vi "Get Status.vi"(7 "Server Alias":string, 8 "error in (no error)":errorcluster, 9 "Clear Status? (F)":bool, 10 "Include Script Status? (T)":bool=TRUE, 11 "Include Timestamps in Script Status? (T)":bool=TRUE) -> (0 "error out":errorcluster, 1 "Script Status":string, 2 "Connected":bool, 4 "All Scripts":T1[](array[typedef]), 5 "Python Just Disconnected":bool, 6 "Index of Last Line":i32)   [LabVIEW 2013, in "TS.lvlib"]
doc: "This VI polls the Server to know the status, whether the LV side is initialized, whether there is a connection with the Python side, and the status of any scripts running."
uses:
  TS.lvlib
  Private/Status Message.ctl
  LabVIEW Example/Supporting Code/Script Running.ctl
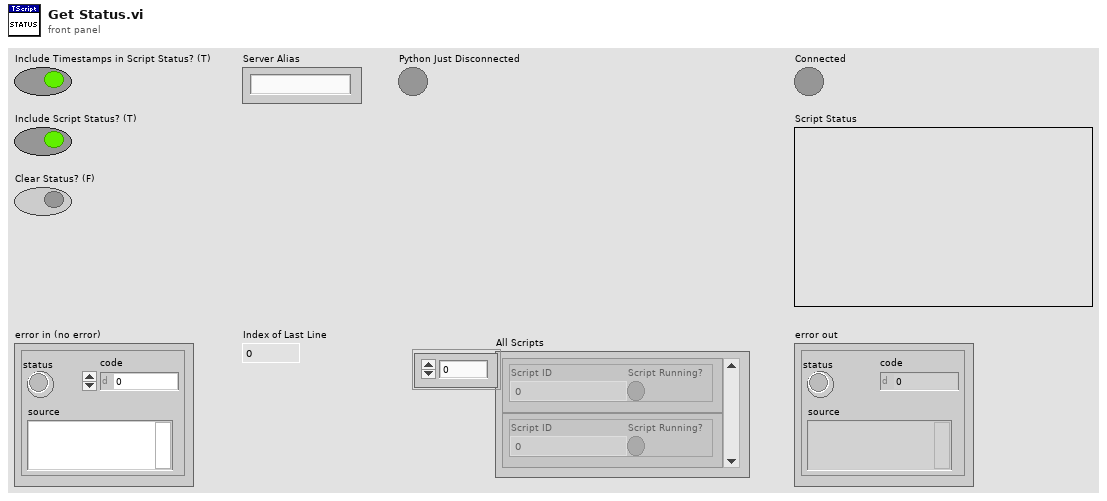
[diagram p1: front panel]
types:
  T1 = typedef "TS.lvlib/Script Running.ctl" = cluster{"Script ID":i64, "Script Running?":bool}
  T2 = typedef "TS.lvlib/Status Message.ctl" = cluster{"Text":string, "Time":timestamp}
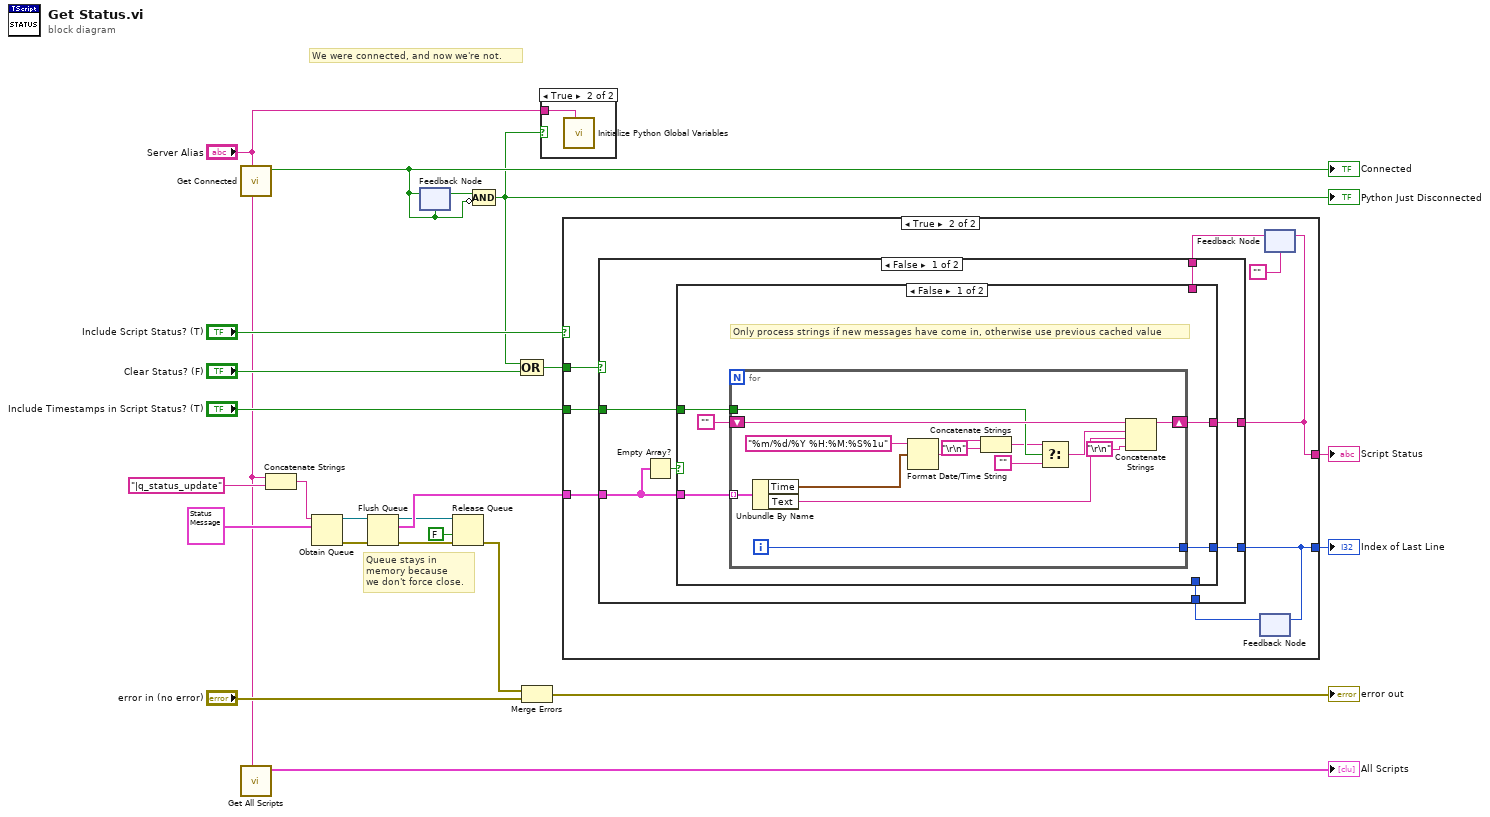
[diagram p0: block diagram]
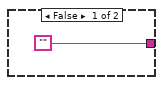
[diagram p3: hidden frame]
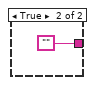
[diagram p5: hidden frame]
diagram:
  # "Queue stays in \nmemory because\nwe don't force close."
  # "We were connected, and now we're not."
  n1 = call "Get Connected.vi"("Server Alias"="Server Alias") -> ("Connected"=w4:bool)  [unwired: 9 in, 1 out]
  "Connected" <- w4
  n2 = call "Get All Scripts.vi"("Server Alias"="Server Alias") -> ("All Scripts"=→"All Scripts":T1[])  [unwired: 9 in, 1 out]
  n3 = Concatenate Strings("Server Alias", "|q_status_update" ("name (unnamed)")) -> (w3:string)
  n4 = Obtain Queue(name (unnamed)=w3, element data type=T2 {"Text"="", "Time"=timestamp(0 s since 1904-01-01)} ("Status Update Message")) -> (queue out=w12:refnum<queue>, error out=w11:errorcluster)  [unwired: 3 in, 1 out]
  n5 = Flush Queue(queue=w12, error in (no error)=w11) -> (queue out=w9:refnum<queue>, remaining elements=w18:T2[], error out=w10:errorcluster)
  n6 = feedback-in #1(w4) -> ()
  n7 = feedback #1(w4) -> (w17:bool)
  n8 = Release Queue(queue=w9, force destroy? (F)=FALSE, error in (no error)=w10) -> (error out=w6:errorcluster)  [unwired: 2 out]
  n9 = Compound Arithmetic op=AND(w17, invert w4) -> (w2:bool)
  "Python Just Disconnected" <- w2
  n10 = Compound Arithmetic op=OR(w2, "Clear Status? (F)") -> (w16:bool)
  n11 = Merge Errors(w6, "error in (no error)") -> (→"error out":errorcluster)
  n12 = case shown="True" w2 {
    tunnel: "Server Alias" -> [_ w24]
    frame False {
    }
    frame True {
      n13 = call "Initialize Python Global Variables.vi"("Server Alias"=w24) -> ()  [unwired: 10 in, 1 out]
    }
  }
  n14 = case shown="True" "Include Script Status? (T)" {
    tunnel: "Include Timestamps in Script Status? (T)" -> [_ w29]
    tunnel: ["" ("Script Status") w33] -> w20
    tunnel: [_ w31] -> w19
    tunnel: w16 -> [_ w27]
    tunnel: w18 -> [_ w28]
    frame False {
    }
    frame True {
      n15 = feedback #2() -> (w30:i32)  [unwired: 1 in]
      n16 = feedback #3("") -> (w32:string)
      n17 = case shown="False" w27 {
        tunnel: [w40 ""] -> w33
        tunnel: w32 -> [w39 _]
        tunnel: [w38 _] -> w31
        tunnel: w30 -> [w37 _]
        tunnel: w29 -> [w35 _]
        tunnel: w28 -> [w34 _]
        frame False {
          n18 = Empty Array?(array=w34) -> (empty?=w36:bool)
          n19 = case shown="False" w36 {
            tunnel: [w44 w60] -> w40
            tunnel: [w43 w61] -> w38
            tunnel: w39 -> [_ w60]
            tunnel: w37 -> [_ w61]
            tunnel: w34 -> [w42 _]
            tunnel: w35 -> [w41 _]
            frame False {
              # "Only process strings if new messages have come in, otherwise use previous cached value"
              n20 = for {
                tunnel: w41 -> [w51]
                shift-right: [w58] -> w44
                shift-left: "" -> [w57]
                tunnel: [w56] -> w43
                tunnel: w42 -> [w55] mode=indexing
                i -> [w56]
                n21 = Unbundle By Name(w55) -> ("Time"=w53:timestamp, "Text"=w52:string)
                n22 = Format Date/Time String(time format string (%c)="%m/%d/%Y %H:%M:%S%1u", seconds (now)=w53) -> (date/time string=w49:string)  [unwired: 1 in]
                n23 = Concatenate Strings(w49, "\r\n") -> (w48:string)
                n24 = Select(t=w48, s=w51, f="") -> (s? t:f=w46:string)
                n25 = Concatenate Strings(w57, w46, w52, "\r\n") -> (w58:string)
              }
            }
            frame True {
            }
          }
        }
        frame True {
        }
      }
      n26 = feedback-in #2(w31) -> ()
      n27 = feedback-in #3(w33) -> ()
    }
  }
  "Script Status" <- w20
  "Index of Last Line" <- w19
